vi "Percent Decode.vi"(1 "escaped string in":string) -> (0 "unescaped string out":string)   [LabVIEW 2011, in "i3-oauth.lvlib"]
doc: "Percent decodes the provided string. Assumes that all percent signs are associated with percent encoded characters."
uses:
  i3-oauth.lvlib
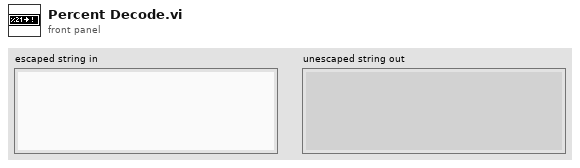
[diagram p1: front panel]
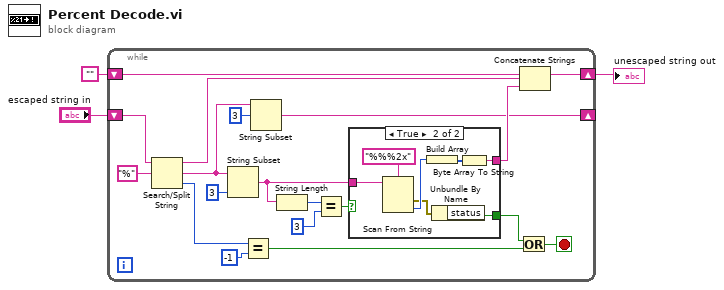
[diagram p0: block diagram]
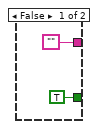
[diagram p2: hidden frame]
diagram:
  n1 = while {
    shift-right: [w21] -> w3
    shift-left: "" -> [w22]
    shift-right: [w4] -> _
    shift-left: "escaped string in" -> [w20]
    stop <- w10 stop-if-true
    n2 = Search/Split String(string=w20, search string/char (-)="%") -> (substring before match=w18:string, match + rest of string=w5:string, offset of match=w7:i32)  [unwired: 1 in]
    n3 = String Subset(string=w5, length (rest)=3 ("length (rest)")) -> (substring=w13:string)  [unwired: 1 in]
    n4 = Equal?(x=w7, y=-1) -> (x = y?=w9:bool)
    n5 = String Subset(string=w5, offset (0)=3 ("length (rest)")) -> (substring=w4:string)  [unwired: 1 in]
    n6 = String Length(string=w13) -> (length=w16:i32)
    n7 = Equal?(x=w16, y=3) -> (x = y?=w14:bool)
    n8 = case shown="True" w14 {
      tunnel: w13 -> [_ w31]
      tunnel: [TRUE ("status") w26] -> w8
      tunnel: ["" w25] -> w12
      frame False {
      }
      frame True {
        n9 = Scan From String(format string="%%%2x", input string=w31) -> (error out=w27:errorcluster, output 1=w29:i32)  [unwired: 3 in, 2 out]
        n10 = Build Array(w29) -> (w28:i32[])
        n11 = Unbundle By Name(w27) -> ("status"=w26:bool)
        n12 = Byte Array To String(unsigned byte array=w28) -> (string=w25:string)
      }
    }
    n13 = Or(x=w8, y=w9) -> (x .or. y?=w10:bool)
    n14 = Concatenate Strings(w22, w18, w12) -> (w21:string)
  }
  "unescaped string out" <- w3
